vi "StringArray2Binary.vi"(5 "Array in":string[](array[string])) -> (2 "Array out":bool[](array[boolean]))   [LabVIEW 2025]
doc: "Converts 1D array of 0,1 string into Binary Array"
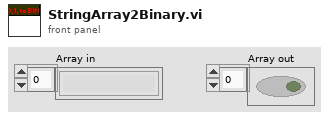
[diagram p1: front panel]
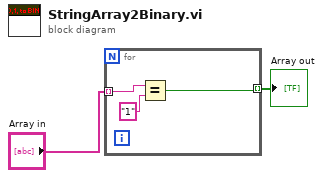
[diagram p0: block diagram]
diagram:
  n1 = for {
    tunnel: "Array in" -> [w5] mode=indexing
    tunnel: [w3] -> w2 mode=indexing
    n2 = Equal?(x=w5, y="1") -> (x = y?=w3:bool)
  }
  "Array out" <- w2
